vi "Init.vi"(6 "Name":string, 9 "Name Library File Path":path, 10 "Type":T1) -> (3 "Name Specs out":refnum<class "Name Specs.lvclass">)   [LabVIEW 2025, in "_Shared.lvlib" / "Name Specs.lvclass"]
uses:
  Name Specs.lvclass
  Type.ctl
  Name Stuff.ctl
  Name Specs.lvclass/Name Specs.ctl
  _Shared.lvlib
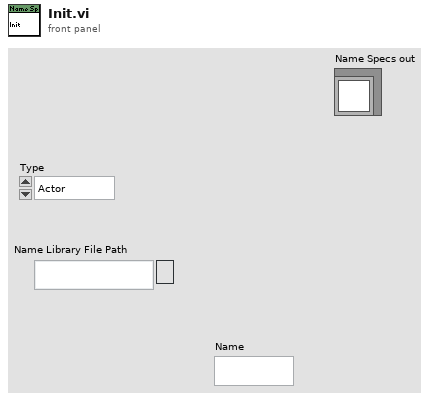
[diagram p1: front panel]
types:
  T1 = typedef "_Shared.lvlib/Type.ctl" = enum16{"Actor", "Msg"}
  T2 = typedef "_Shared.lvlib/Name Stuff.ctl" = cluster{"Type (Enum)":T1, "Type (String)":string, "Name Library File Path":path, "Name":string, "Name Type":string}
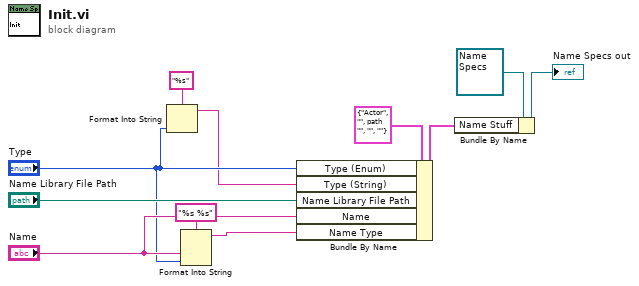
[diagram p0: block diagram]
diagram:
  n1 = Format Into String(format string="%s", "Type") -> (resulting string=w5:string)  [unwired: 2 in, 1 out]
  n2 = Format Into String(format string="%s %s", "Name", "Type") -> (resulting string=w8:string)  [unwired: 2 in, 1 out]
  n3 = Bundle By Name(cluster=T2 {"Type (Enum)"=enum."Actor", "Type (String)"="", "Name Library File Path"=path "", "Name"="", "Name Type"=""} ("Name Stuff"), "Type (Enum)"="Type", "Type (String)"=w5, "Name Library File Path"="Name Library File Path", "Name"="Name", "Name Type"=w8) -> (w1:T2)
  n4 = Bundle By Name(cluster=refnum<class "Name Specs.lvclass"> refnum ("Name Specs in"), "Name Stuff"=w1) -> (→"Name Specs out":refnum<class "Name Specs.lvclass">)
